vi "AddConstantCurrent.vi"(0 "deviceName":string, 1 "channel":u8, 2 "repeats":u16=1, 3 "current":sgl, 4 "samplingInterval":sgl, 5 "maxDuration":sgl, 6 "minSamplingVoltageDifference":sgl=-inf, 7 "error in (no error)":errorcluster, 8 "maxVoltage":sgl=inf, 9 "minVoltage":sgl=-inf, 10 "maxCapacity":sgl=inf, 11 "approxMaxCurrent":sgl=0.1, 12 "isAutoRange":bool=TRUE, 13 "approxMaxVoltage":sgl=0.1, 14 "isAutoVoltageRange":bool=TRUE) -> (27 "error out":errorcluster)   [LabVIEW 2018]
doc: "EXPORT void AisAddConstantCurrent(const char* deviceName, uint8_t channel, uint16_t repeats, float current, float samplingInterval, float maxDuration, float minSamplingVoltageDifference, float maxVoltage, float minVoltage, float maxCapacity, float approxMaxCurrent, bool isAutoRange, float approxMaxVoltage, bool isAutoVoltageRange);"
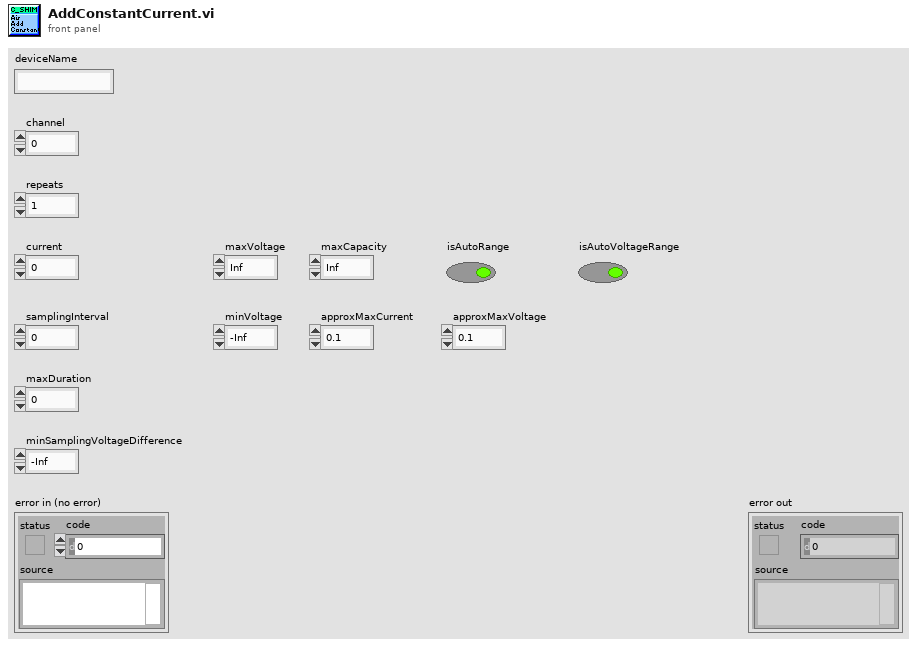
[diagram p1: front panel]
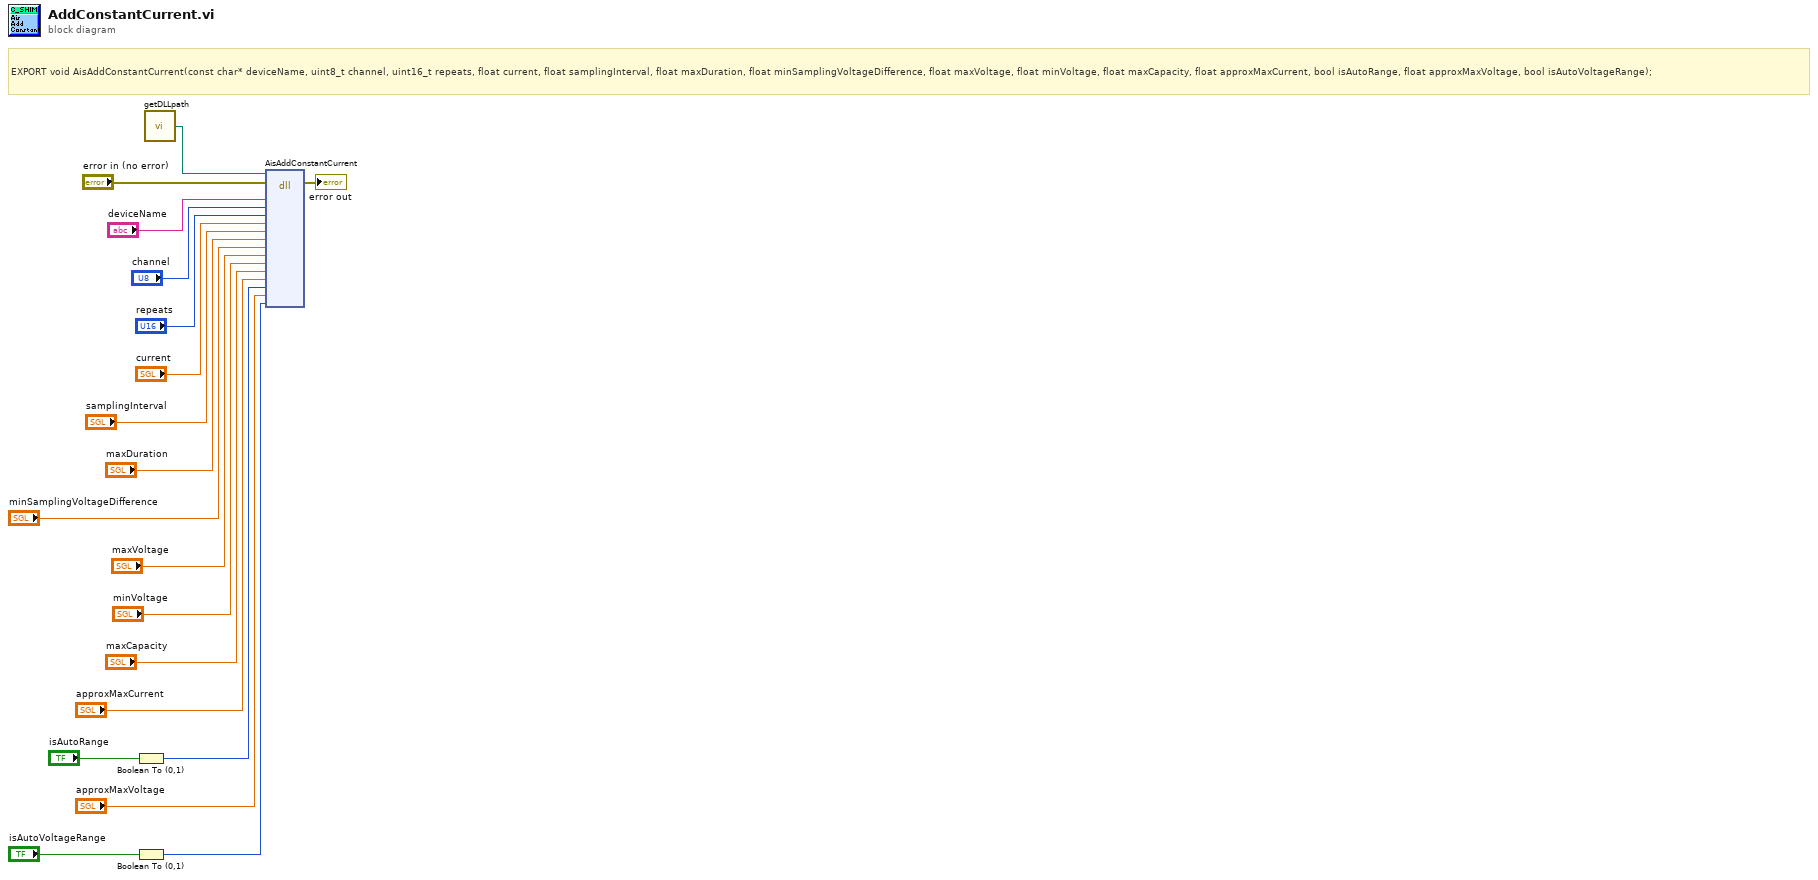
[diagram p0: block diagram]
diagram:
  # "EXPORT void AisAddConstantCurrent(const char* deviceName, uint8_t channel, uint16_t repeats, float current, float samplingInterval, float maxDuration, float minSamplingVoltageDifference, float maxVoltage, float minVoltage, float maxCapacity, float approxMaxCurrent, bool isAutoRange, float approxMaxVoltage, bool isAutoVoltageRange);"
  n1 = Boolean To (0,1)(Boolean="isAutoRange") -> (0, 1=w7:i16)
  n2 = Boolean To (0,1)(Boolean="isAutoVoltageRange") -> (0, 1=w4:i16)
  n3 = call "getDLLpath.vi"() -> ("DLL_Path"=w1:path)
  n4 = dll-call lib="?" fn="AisAddConstantCurrent"(path in=w1, error in="error in (no error)", "deviceName"="deviceName", "channel"="channel", "repeats"="repeats", "current"="current", "samplingInterval"="samplingInterval", "maxDuration"="maxDuration", "minSamplingVoltageDifference"="minSamplingVoltageDifference", "maxVoltage"="maxVoltage", "minVoltage"="minVoltage", "maxCapacity"="maxCapacity", "approxMaxCurrent"="approxMaxCurrent", "isAutoRange"=w7, "approxMaxVoltage"="approxMaxVoltage", "isAutoVoltageRange"=w4) -> (error out=→"error out":errorcluster)  [unwired: 16 in, 1 out]
